vi "例6-12.vi"() -> ()   [LabVIEW 2019]
uses:
  <vilib>/measure/NI_MABase.lvlib
  <vilib>/Analysis/NI_AALPro.lvlib
panel:
  in  "采样点数":dbl=100.0
  in  "采样频率":dbl=100.0
  in  "信号频率":dbl=5.0
  out "相位谱波形":T1(graph)
  out "幅度谱波形":T2(graph)
  out "信号波形":waveform(dbl)(graph)
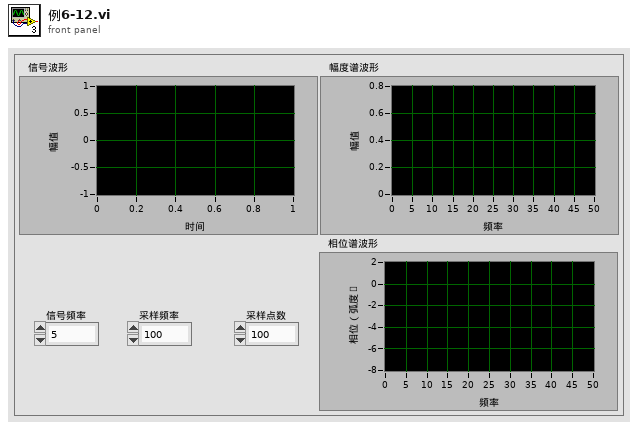
[diagram p1: front panel]
types:
  T1 = cluster{i32, "df":dbl, "Amp Spectrum Phase (radians)":dbl[]}
  T2 = cluster{i32, "df":dbl, "Amp Spectrum Mag (Vrms)":dbl[]}
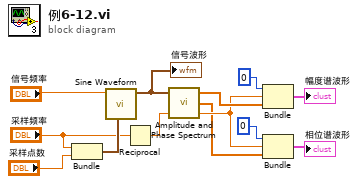
[diagram p0: block diagram]
diagram:
  n1 = Bundle("采样频率"="采样频率", "采样点数"="采样点数") -> (w11:cluster{"采样频率":dbl, "采样点数":dbl})  [unwired: 1 in]
  n2 = call <vilib>:"Sine Waveform.vi"("sampling info"=w11, "frequency"="信号频率") -> ("signal out"=w1:waveform(dbl))  [unwired: 8 in, 1 out]
  "信号波形" <- w1
  n3 = Reciprocal(x="采样频率") -> (1/x=w10:dbl)
  n4 = call <vilib>:"Amplitude and Phase Spectrum.vi"("dt"=w10, "Signal (V)"=w1) -> ("df"=w5:dbl, "Amp Spectrum Phase (radians)"=w4:dbl[], "Amp Spectrum Mag (Vrms)"=w7:dbl[])  [unwired: 1 in]
  n5 = Bundle(0, "df"=w5, "Amp Spectrum Mag (Vrms)"=w7) -> (→"幅度谱波形":T2)  [unwired: 1 in]
  n6 = Bundle(0, "df"=w5, "Amp Spectrum Phase (radians)"=w4) -> (→"相位谱波形":T1)  [unwired: 1 in]
